vi "Destroy.vi"(8 "error in (no error)":errorcluster, 11 "Robot_Interface in":refnum<class "Robot_Interface.lvclass">) -> (0 "error out":errorcluster, 3 "Robot_Interface out":refnum<class "Robot_Interface.lvclass">)   [LabVIEW 2015, in "Robot_Interface.lvclass"]
uses:
  Robot_Interface.lvclass
  Robot_Interface.lvclass/Robot_Interface.ctl
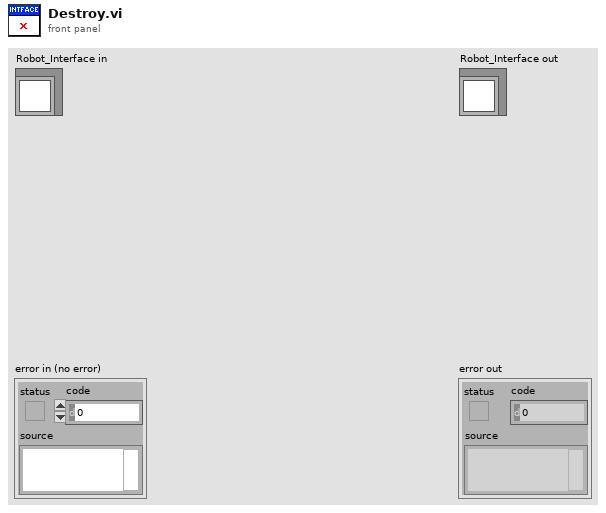
[diagram p1: front panel]
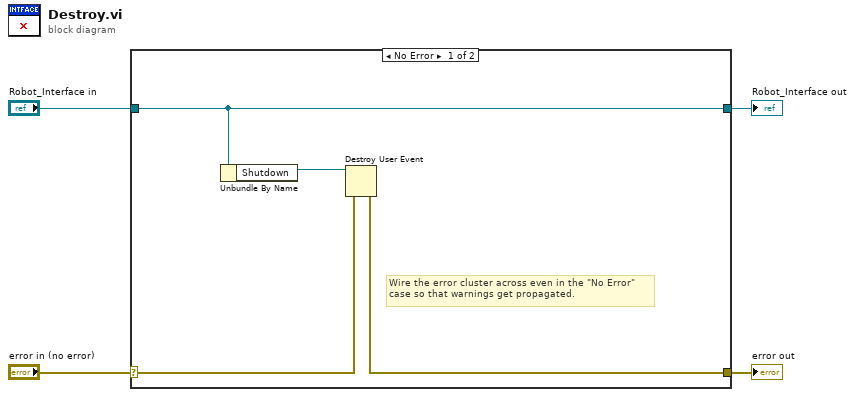
[diagram p0: block diagram]
diagram:
  n1 = case shown="No Error" "error in (no error)" {
    selector: "error in (no error)" -> [w6 w10]
    tunnel: [w5 w10] -> w3
    tunnel: [w8 w9] -> w1
    tunnel: "Robot_Interface in" -> [w8 w9]
    frame No Error {
      # "Wire the error cluster across even in the \"No Error\"\ncase so that warnings get propagated."
      n2 = Unbundle By Name(w8) -> ("Shutdown"=w7:refnum<user-event>)
      n3 = Destroy User Event(user event=w7, error in=w6) -> (error out=w5:errorcluster)
    }
    frame Error {
    }
  }
  "error out" <- w3
  "Robot_Interface out" <- w1
